vi "Read-all-variables.vi"(8 "error in (no error)":errorcluster, 11 "Mapping params. ref. in":refnum<data-value>) -> (0 "error out":errorcluster, 2 "Mapping vars.":T1, 3 "Mapping params. ref.":refnum<data-value>)   [LabVIEW 2013, in "CameraVision.lvlib" / "CV-Mapping.lvclass"]
uses:
  CV-Mapping.lvclass
  Mapping-variables.ctl
  UI/Module-states.ctl
  Mapping-characteristic.ctl
  CV-Mapping.lvclass/CV-Mapping.ctl
  UI/CV-UI.lvclass
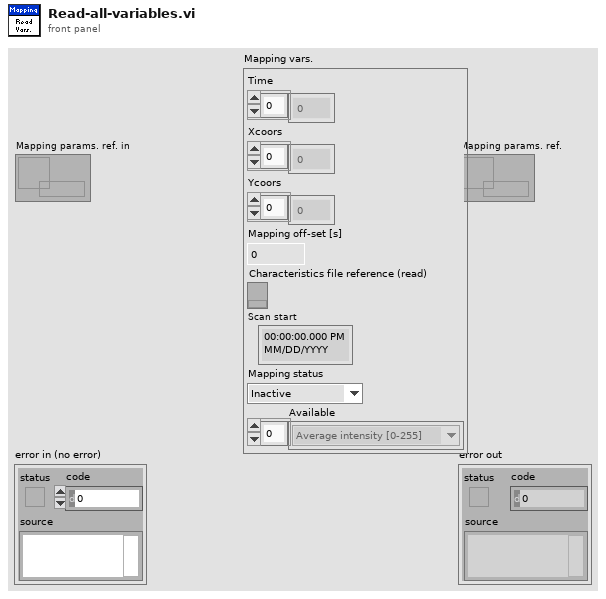
[diagram p1: front panel]
types:
  T1 = typedef "CameraVision.lvlib/CV-Mapping.lvclass/Mapping-variables.ctl" = cluster{"Time":sgl[], "Xcoors":sgl[], "Ycoors":sgl[], "Mapping off-set":dbl, "Characteristics file reference (read)":refnum<k34>, "Scan start":timestamp, "Mapping status":T2, "Available":T3[]}
  T2 = typedef "CameraVision.lvlib/CV-UI.lvclass/Module-states.ctl" = enum16{"Inactive", "Active", "Data-loss", "Error", "Simulation", "Synchronizing", "Initialized", "Released"}
  T3 = typedef "CameraVision.lvlib/CV-Mapping.lvclass/Mapping-characteristic.ctl" = enum16{"Average intensity [0-255]", "Peak intensity [0-255]", "Melt-pool size [mm²]", "Melt-pool aspect ratio []", "Melt-pool fragments []", "Average temperature [°C]", "Max. temperature [°C]", "Min. temperature [°C]", "Std. dev. temperature [°C]"}
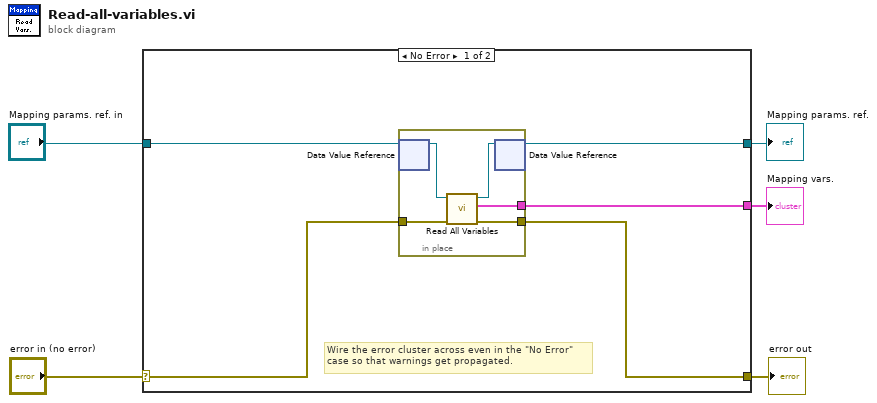
[diagram p0: block diagram]
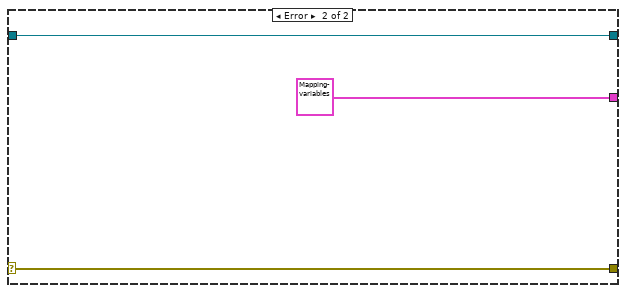
[diagram p2: hidden frame]
diagram:
  n1 = case shown="No Error" "error in (no error)" {
    selector: "error in (no error)" -> [w8 w18]
    tunnel: [w10 w18] -> w4
    tunnel: "Mapping params. ref. in" -> [w7 w16]
    tunnel: [w9 T1 {"Time"=[], "Xcoors"=[], "Ycoors"=[], "Mapping off-set"=0.0, "Characteristics file reference (read)"=refnum, "Scan start"=timestamp(0 s since 1904-01-01), "Mapping status"=enum."Inactive", "Available"=[]} ("Mapping vars.")] -> w2
    tunnel: [w6 w16] -> w1
    frame No Error {
      # "Wire the error cluster across even in the \"No Error\"\ncase so that warnings get propagated."
      n2 = in-place {
        in-place-border: [w15] -> w10
        in-place-border: [w14] -> w9
        in-place-border: w8 -> [w13]
        n3 = in-place-dvr #1(w7) -> (w11:refnum<class "CV-Mapping.lvclass">)  [unwired: 1 out]
        n4 = call "Read All Variables.vi"("error in (no error)"=w13, "Mapping params in"=w11) -> ("error out"=w15:errorcluster, "Mapping vars."=w14:T1, "Mapping params out"=w12:refnum<class "CV-Mapping.lvclass">)  [unwired: 7 in]
        n5 = in-place-dvr #1(w12) -> (w6:refnum<data-value>)  [unwired: 1 out]
      }
    }
    frame Error {
    }
  }
  "error out" <- w4
  "Mapping params. ref." <- w1
  "Mapping vars." <- w2
